vi "LV Exp8.vi"() -> ()   [LabVIEW 2009]
uses:
  <vilib>/NXT/Block Support/NXT_InputPort.ctl
  <vilib>/NXT/Dual Mode Library/Waits/Wait_Num(msec).vi
  <vilib>/NXT/Dual Mode Library/Display/drawText.vi
panel:
  out "Temperature":sgl
  in  "Threshold":sgl=23.0
  in  "stop":bool
  out "LED":bool
  out "Message":string
  # "HiTechnic Experimenter's Kit\n\n                        Experiment 8 - Temperature Sensor\nThis program reads the temperature chip on A0 and calculate the temperature in degrees C.  Turn on the LED connected to  B4 if the temperature is above set value.\n\nSee Experimenter's Kit Handbook for the SuperPro for\nmore information or go to www.hitechnic.com.\n\n(c) HiTechnic 2011"
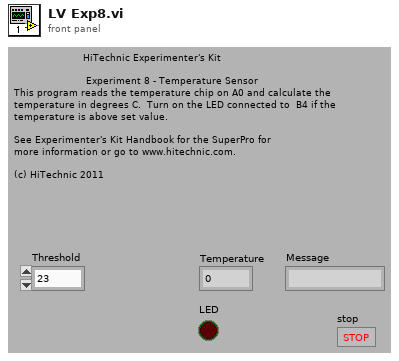
[diagram p1: front panel]
types:
  T1 = typedef "NXT_InputPort.ctl" = u8
  T2 = typedef "LVHSConnector.ctl" = cluster{"error":errorcluster, "address":string, "NXT #":i32, "Show Error":bool, "Connection":u16}
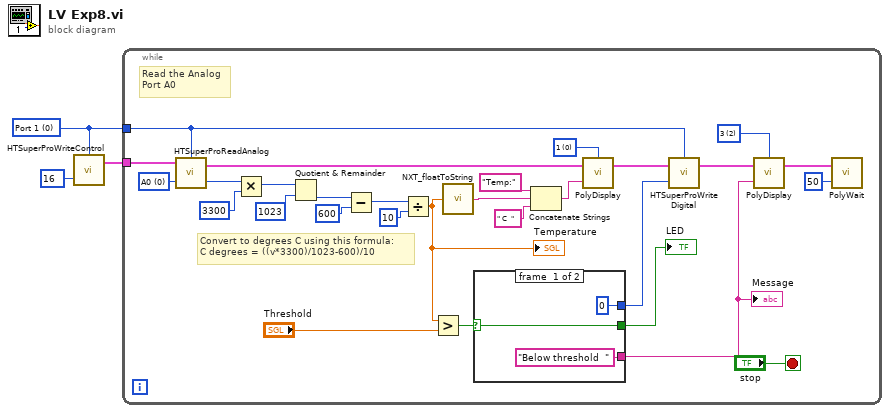
[diagram p0: block diagram]
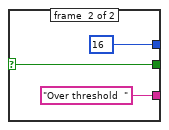
[diagram p2: hidden frame]
diagram:
  w1 = T1 0 items=["Port 1", "Port 2", "Port 3", "Port 4"] ("Port")
  n1 = call "HTSuperProWriteControl.vi"("Digital Value"=u8 16, "Port"=w1) -> ("NXT"=w3:T2)  [unwired: 3 in]
  n2 = while {
    tunnel: w1 -> [w31]
    tunnel: w3 -> [w32]
    stop <- "stop" stop-if-true
    w9 = i16 0 items=["1", "2", "3", "4", "5", "6", "7", "8"] ("Line")
    w27 = u8 0 items=["A0", "A1", "A2", "A3"] ("Analog Port")
    w28 = i16 2 items=["1", "2", "3", "4", "5", "6", "7", "8"] ("Line")
    # "Convert to degrees C using this formula:\nC degrees = ((v*3300)/1023-600)/10"
    # "Read the Analog\nPort A0"
    n3 = call "HTSuperProReadAnalog.vi"("Analog Port"=w27, "NXT"=w32, "Port"=w31) -> ("Analog Value"=w26:i16, "NXT"=w13:T2)  [unwired: 1 in]
    n4 = Multiply(x=w26, y=3300) -> (x*y=w24:i32)
    n5 = Quotient & Remainder(x=w24, y=1023) -> (floor(x/y)=w22:i32)  [unwired: 1 out]
    n6 = Subtract(x=w22, y=600) -> (x-y=w20:i32)
    n7 = Divide(x=w20, y=10) -> (x/y=w5:dbl)
    "Temperature" <- w5
    n8 = Greater?(x=w5, y="Threshold") -> (0:w18:bool)
    n9 = call <vilib>:"NXT_floatToString.vi"("number"=w5) -> ("string"=w6:string)
    n10 = case shown="True" w18 {
      selector: w18 -> [w34 w38]
      tunnel: [w34 w38] -> w17
      tunnel: [u8 0 ("Digital Value") u8 16 ("Digital Value")] -> w16
      tunnel: ["Below threshold  " "Over threshold  "] -> w15
      frame #0 {
      }
      frame #1 {
      }
    }
    "LED" <- w17
    "Message" <- w15
    n11 = Concatenate Strings("Temp:" ("string"), w6, " C  " ("string")) -> (w12:string)
    n12 = call-poly <vilib>:"PolyDisplay.vi"("Text"=w12, "NXT"=w13, "Line"=w9) -> ("NXT"=w14:T2)  [unwired: 1 in]
    n13 = call "HTSuperProWriteDigital.vi"("Digital Value"=w16, "NXT"=w14, "Port"=w31) -> ("NXT"=w29:T2)  [unwired: 2 in]
    n14 = call-poly <vilib>:"PolyDisplay.vi"("Text"=w15, "NXT"=w29, "Line"=w28) -> ("NXT"=w8:T2)  [unwired: 1 in]
    n15 = call-poly <vilib>:"PolyWait.vi"("Time (100 msec)"=u32 50 ("Time (1 sec)"), "NXT"=w8) -> ()  [unwired: 2 in, 1 out]
  }
